vi "Field Draw Targets.vi"(4 "Lado":enum16{"Esquerdo", "Direito"}(ring) caption="Enum", 6 "Draw Targets?":T1, 8 "Picture In":picture, 9 "Offset":cluster{"Width":dbl, "Height":dbl}, 10 "Scale":dbl, 11 "our_robots":T2[](array[typedef])) -> (0 "Picture Out":picture, 1 "Offset Out":cluster{"Width":dbl, "Height":dbl}, 2 "Scale Out":dbl)   [LabVIEW 2017]
uses:
  Core/AI Robot.ctl
  Intel/Functions Enum.ctl
  Intel/AttackerStates.ctl
  DrawTargets.ctl
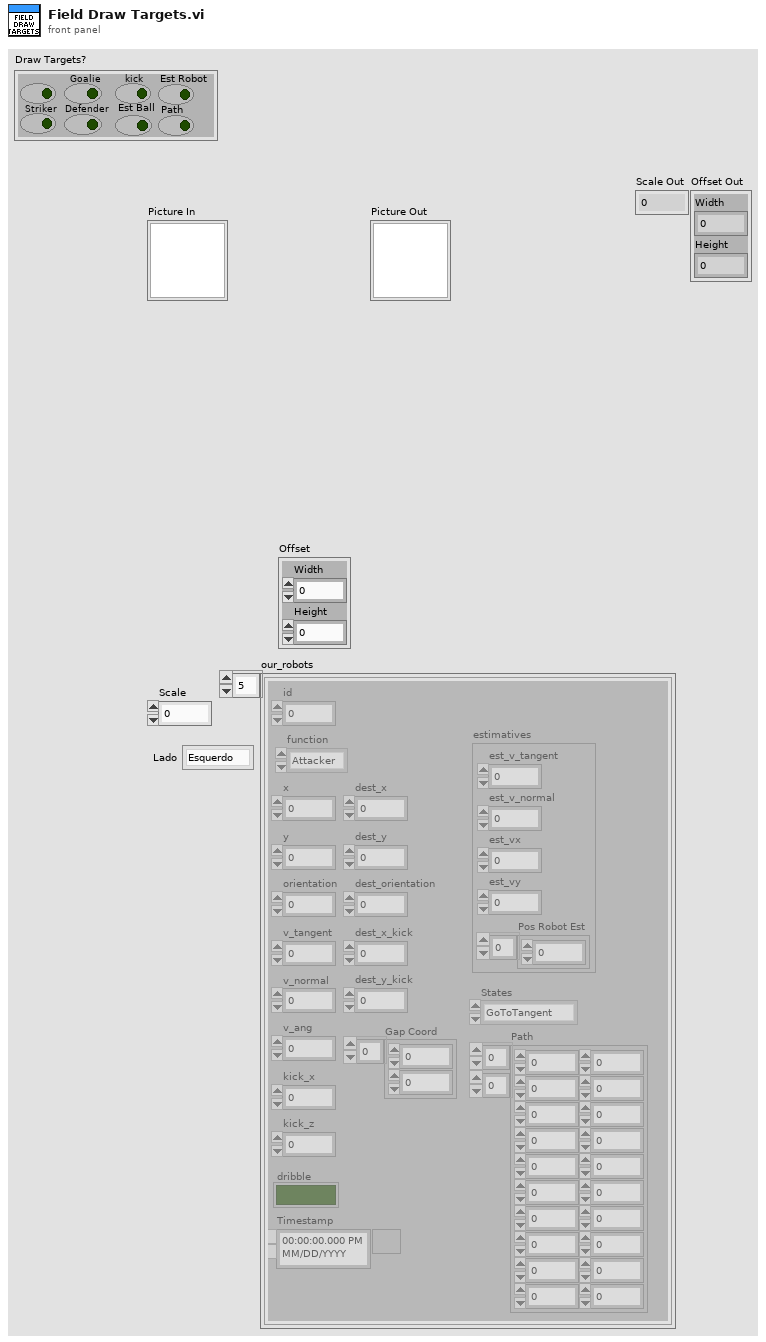
[diagram p1: front panel]
types:
  T1 = typedef "DrawTargets.ctl" = cluster{"Attacker":bool, "Striker":bool, "Goalie":bool, "Defender":bool, "kick":bool, "Est Ball":bool, "Est Robot":bool, "Path":bool}
  T2 = typedef "AI Robot.ctl" = cluster{"id":u32, "function":T3, "x":dbl, "y":dbl, "orientation":dbl, "v_tangent":dbl, "v_normal":dbl, "v_ang":dbl, "kick_x":dbl, "kick_z":dbl, "dribble":bool, "Timestamp":timestamp, "dest_x":dbl, "dest_y":dbl, "dest_orientation":dbl, "estimatives":cluster{"est_v_tangent":dbl, "est_v_normal":dbl, "est_vx":dbl, "est_vy":dbl, "Pos Robot Est":dbl[]}, "dest_x_kick":dbl, "dest_y_kick":dbl, "Gap Coord":dbl[], "States":T4, "Path ":dbl[][]}
  T3 = typedef "Functions Enum.ctl" = enum16{"Attacker", "Goalie", "Defender", "Striker", "Goto 0", "Dummy", "Kicker", "ZigZag"}
  T4 = typedef "AttackerStates.ctl" = enum16{"Pass", "GoToTangent", "BallGetting", "GoToKick", ""}
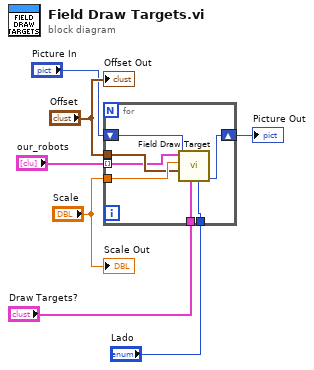
[diagram p0: block diagram]
diagram:
  n1 = for {
    tunnel: "Scale" -> [w14]
    tunnel: "Offset" -> [w12]
    shift-right: [w13] -> w4
    shift-left: "Picture In" -> [w11]
    tunnel: "our_robots" -> [w10] mode=indexing
    tunnel: "Draw Targets?" -> [w9]
    tunnel: "Lado" -> [w8]
    n2 = call "Field Draw Target.vi"("Lado"=w8, "Draw Targets?"=w9, "picture in"=w11, "Offset"=w12, "Scale mm/pixel"=w14, "Robot"=w10) -> ("picture out"=w13:picture)  [unwired: 5 in]
  }
  "Picture Out" <- w4
  "Scale Out" <- "Scale"
  "Offset Out" <- "Offset"
